vi "Write Vsp.vi"(8 "error in (no error)":errorcluster, 10 "Vsp":dbl, 11 "Session HVPS in":refnum<class "Session HVPS.lvclass">) -> (0 "error out":errorcluster, 3 "Session HVPS out":refnum<class "Session HVPS.lvclass">)   [LabVIEW 2014, in "Session HVPS.lvclass"]
uses:
  Session HVPS.lvclass
  Session HVPS.lvclass/Session HVPS.ctl
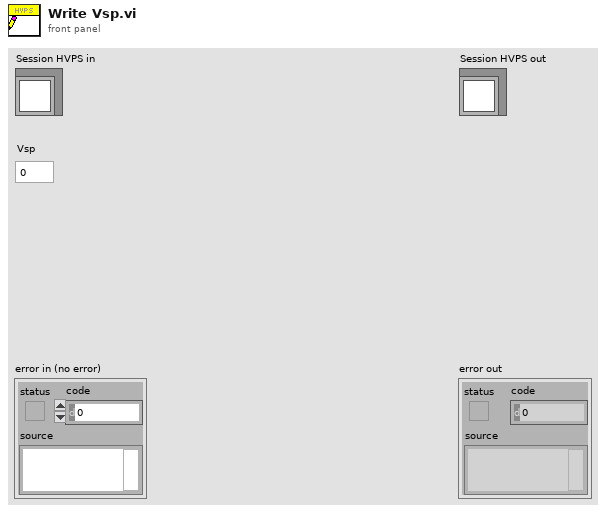
[diagram p1: front panel]
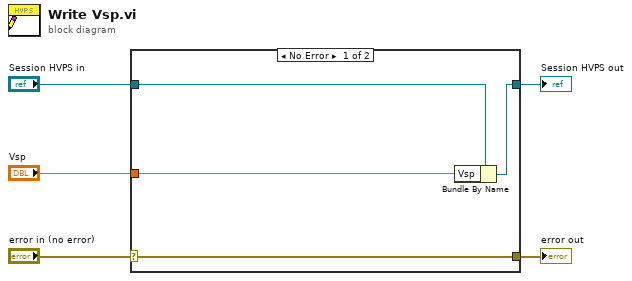
[diagram p0: block diagram]
diagram:
  n1 = case shown="No Error" "error in (no error)" {
    selector: "error in (no error)" -> [w9 w10]
    tunnel: [w9 w10] -> w4
    tunnel: [w7 w11] -> w2
    tunnel: "Session HVPS in" -> [w8 w11]
    tunnel: "Vsp" -> [w6 _]
    frame No Error {
      n2 = Bundle By Name(cluster=w8, "Vsp"=w6) -> (w7:refnum<class "Session HVPS.lvclass">)
    }
    frame Error {
    }
  }
  "error out" <- w4
  "Session HVPS out" <- w2
